vi "Write Schema.vi"(8 "error in (no error)":errorcluster, 10 "Schema":string, 11 "Import Export in":refnum<class "Import Export SQL.lvclass">) -> (0 "error out":errorcluster, 3 "Import Export out":refnum<class "Import Export SQL.lvclass">)   [LabVIEW 2023, in "Data Analysis.lvlib" / "Import Export SQL.lvlib" / "Import Export SQL.lvclass"]
uses:
  Import Export SQL.lvclass
  Import Export SQL.lvclass/Import Export SQL.ctl
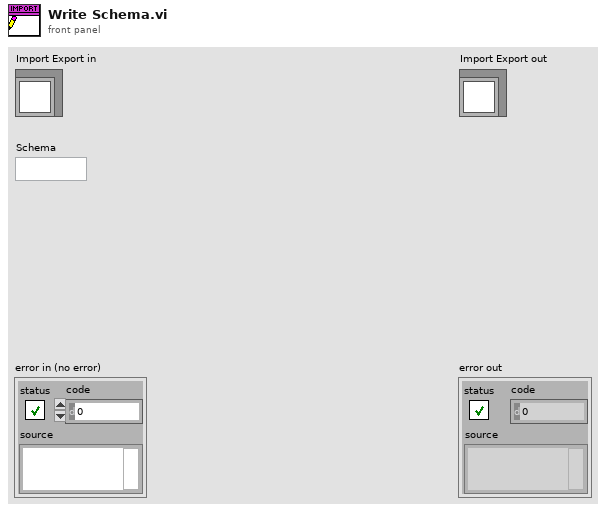
[diagram p1: front panel]
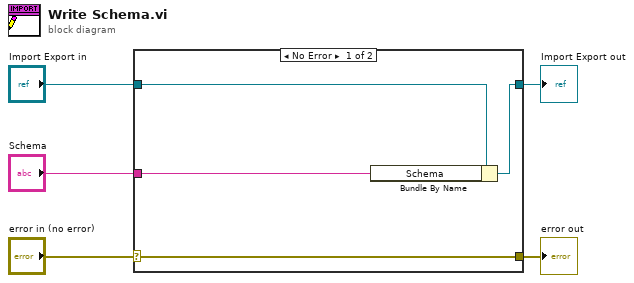
[diagram p0: block diagram]
diagram:
  n1 = case shown="No Error" "error in (no error)" {
    selector: "error in (no error)" -> [w9 w10]
    tunnel: [w9 w10] -> w4
    tunnel: [w7 w11] -> w2
    tunnel: "Import Export in" -> [w8 w11]
    tunnel: "Schema" -> [w6 _]
    frame No Error {
      n2 = Bundle By Name(cluster=w8, "Schema"=w6) -> (w7:refnum<class "Import Export SQL.lvclass">)
    }
    frame Error {
    }
  }
  "error out" <- w4
  "Import Export out" <- w2
